vi "Configure Sys (To) AutoRun.vi"(8 "error in (no error)":errorcluster, 10 "AutoRun (F:Disabled)":bool, 11 "VISA resource name":refnum<visa-resource-name>) -> (0 "error out":errorcluster, 3 "VISA resource name out":refnum<visa-resource-name>)   [LabVIEW 2012, in "Quantum Composers 9000 Series.lvlib"]
doc: "This VI is used to enable/disable the auto-run feature. If auto-run is enabled, pulse generation begins when the unit is powered on.\n\nValid Range:\nT: Enabled\nF: Disabled (default)"
uses:
  <instrlib>/Quantum Composers 9000 Series/Quantum Composers 9000 Series.lvlib
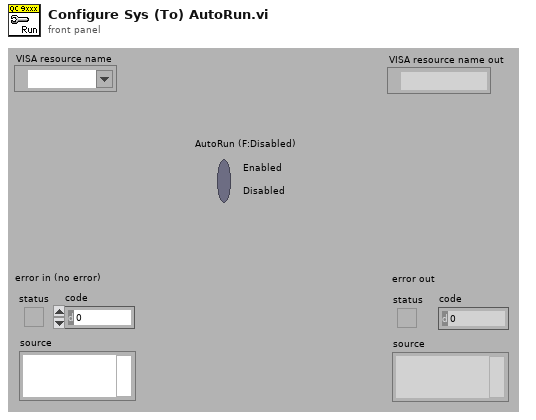
[diagram p1: front panel]
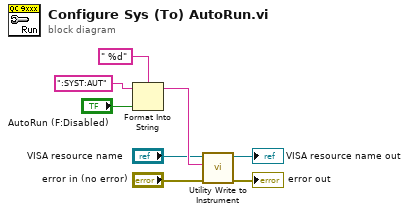
[diagram p0: block diagram]
diagram:
  n1 = Format Into String(format string=" %d", initial string=":SYST:AUT", "AutoRun (F:Disabled)") -> (resulting string=w5:string)  [unwired: 1 in, 1 out]
  n2 = call <instrlib>:"Utility Write to Instrument.vi"("error in (no error)"="error in (no error)", "Write Buffer"=w5, "VISA resource name"="VISA resource name") -> ("error out"=→"error out":errorcluster, "VISA resource name out"=→"VISA resource name out":refnum<visa-resource-name>)  [unwired: 6 in, 1 out]
